vi "Populate Field.vi"(8 "error in (no error)":errorcluster, 10 "Field Name":string, 11 "Panel Form Controller in":refnum<class "Panel Form Controller.lvclass">) -> (0 "error out":errorcluster, 3 "Panel Form Controller out":refnum<class "Panel Form Controller.lvclass">)   [LabVIEW 2020, in "Panel Form Controller.lvlib" / "Panel Form Controller.lvclass"]
uses:
  Panel Form Controller.lvclass
  Panel Form Controller.lvclass/Panel Form Controller.ctl
  source/Field/Field.lvclass
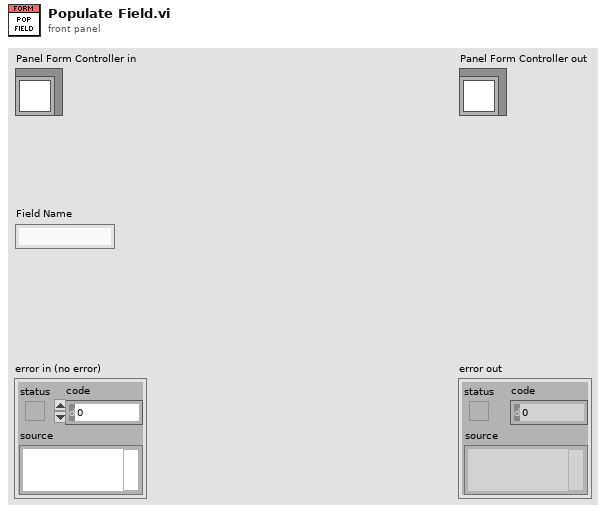
[diagram p1: front panel]
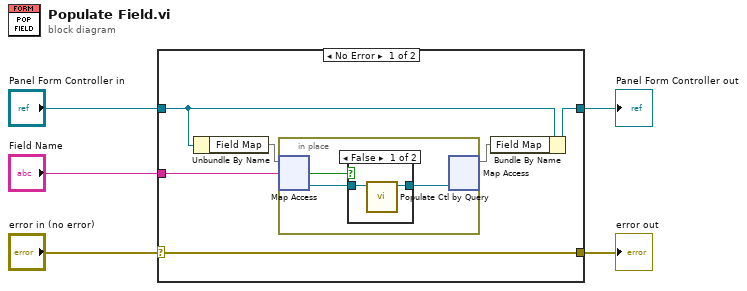
[diagram p0: block diagram]
diagram:
  n1 = case shown="No Error" "error in (no error)" {
    selector: "error in (no error)" -> [w11 w19]
    tunnel: [w11 w19] -> w4
    tunnel: [w9 w18] -> w2
    tunnel: "Panel Form Controller in" -> [w10 w18]
    tunnel: "Field Name" -> [w8 _]
    frame No Error {
      n2 = Unbundle By Name(w10) -> ("Field Map"=w7:map{string, refnum<class "Field.lvclass">})
      n3 = in-place {
        n4 = in-place-map #1(w7, w8) -> (w14:refnum<class "Field.lvclass">, w12:bool)  [unwired: 1 in]
        n5 = case shown="False" w12 {
          tunnel: w14 -> [w16 w17]
          tunnel: [w15 w17] -> w13
          frame False {
            n6 = call-dynamic "Populate Ctl by Query.vi"("Field in"=w16) -> ("Field out"=w15:refnum<class "Field.lvclass">)  [unwired: 9 in, 1 out]
          }
          frame True {
          }
        }
        n7 = in-place-map #1(w13) -> (w6:map{string, refnum<class "Field.lvclass">})  [unwired: 1 in, 2 out]
      }
      n8 = Bundle By Name(cluster=w10, "Field Map"=w6) -> (w9:refnum<class "Panel Form Controller.lvclass">)
    }
    frame Error {
    }
  }
  "error out" <- w4
  "Panel Form Controller out" <- w2
